vi "NewAutoAbsTrajSelector.vi"() -> ()   [LabVIEW 2023]
uses:
  Trajectory/TrajectoryGlobals.vi
panel:
  in  "AbsoluteTrajectoryInput":i32
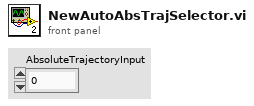
[diagram p1: front panel]
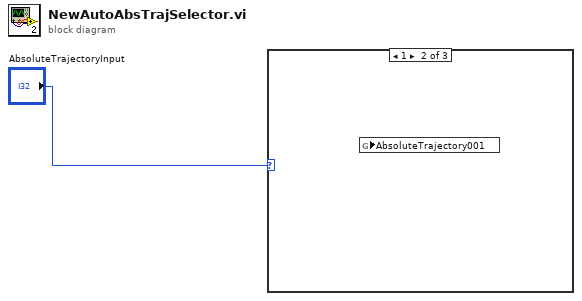
[diagram p0: block diagram]
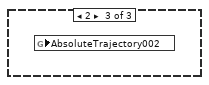
[diagram p3: hidden frame]
diagram:
  n1 = case shown="1" "AbsoluteTrajectoryInput" {
    frame 0, Default {
    }
    frame 1 {
      n2 = global read "TrajectoryGlobals.vi" "AbsoluteTrajectory001"() -> ()  [unwired: 1 in]
    }
    frame 2 {
      n3 = global read "TrajectoryGlobals.vi" "AbsoluteTrajectory002"() -> ()  [unwired: 1 in]
    }
  }
